vi "new_vi.vi"(6 "wait for reply (T)":bool=TRUE, 8 "error in":errorcluster) -> (0 "error out":errorcluster, 1 "timed out?":bool, 2 "result":string, 3 "vi_id":i32)   [LabVIEW 2025, in "Scripting Server.lvlib"]
doc: "Creates a new VI in the LabVIEW IDE. The VI Reference is stored and returned. This Reference can later be used to e.g. add modifications to the VI."
uses:
  Scripting Server.lvlib
  New VI Argument--cluster.ctl
  New VI (Reply Payload)--cluster.ctl
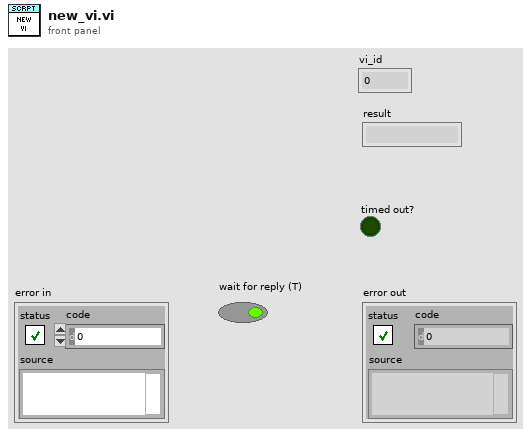
[diagram p1: front panel]
types:
  T1 = typedef "Scripting Server.lvlib/New VI Argument--cluster.ctl" = cluster{"Open Frontpanel":bool, "Wait Notifier":refnum<notifier>, "wait for reply":bool}
  T2 = typedef "Scripting Server.lvlib/Request Events--cluster.ctl" = cluster{"Stop Module":refnum<user-event>, "Show Panel":refnum<user-event>, "Hide Panel":refnum<user-event>, "Get Module Execution Status":refnum<user-event>, "Show Diagram":refnum<user-event>, "New VI":refnum<user-event>, "Add Object":refnum<user-event>, "Connect Objects":refnum<user-event>, "Get Object Terminals":refnum<user-event>, "get vi error list":refnum<user-event>, "Cleanup VI":refnum<user-event>, "create_control":refnum<user-event>, "Run VI":refnum<user-event>}
  T3 = typedef "Scripting Server.lvlib/New VI (Reply Payload)--cluster.ctl" = cluster{"VI Reference":i32, "Result":string, "error":errorcluster}
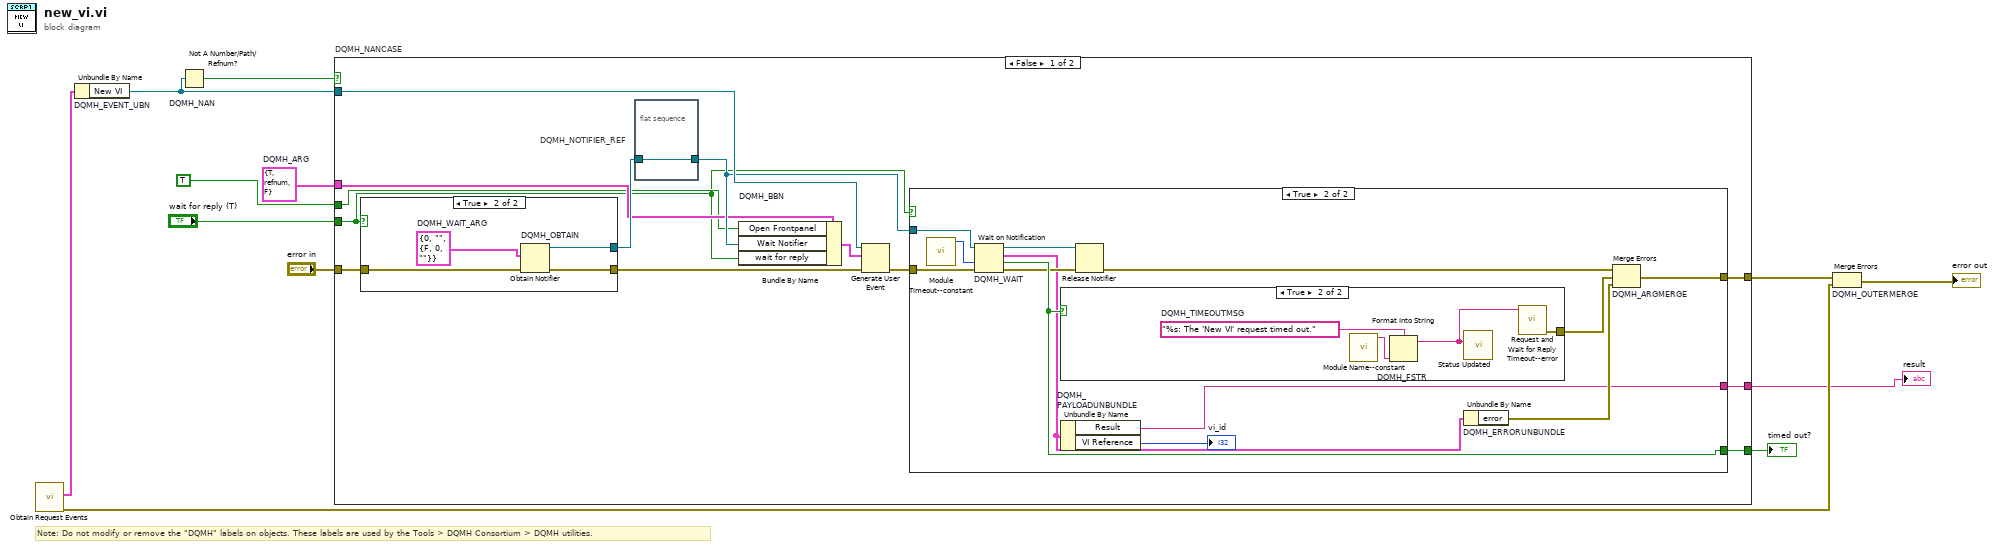
[diagram p0: block diagram]
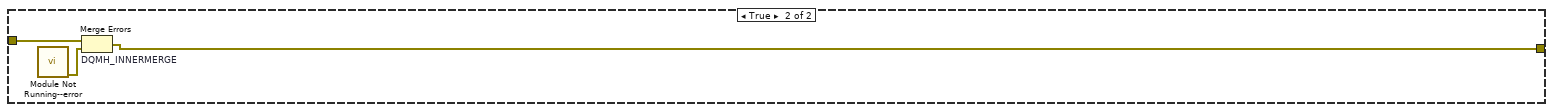
[diagram p5: hidden frame]
diagram:
  w6 = T1 {"Open Frontpanel"=TRUE, "Wait Notifier"=refnum, "wait for reply"=FALSE}  # DQMH_ARG
  # "Note: Do not modify or remove the \"DQMH\" labels on objects. These labels are used by the Tools > DQMH Consortium > DQMH utilities."
  n1 = call "Obtain Request Events.vi"() -> ("error out"=w3:errorcluster, "Scripting Server Request Events"=w2:T2)  [unwired: 10 in]
  n2 = Unbundle By Name "DQMH_EVENT_UBN"(w2) -> ("New VI"=w10:refnum<user-event>)
  n3 = Not A Number/Path/Refnum? "DQMH_NAN"(number/path/refnum=w10) -> (NaN/Path/Refnum?=w9:bool)
  n4 = case "DQMH_NANCASE" shown="False" w9 {
    tunnel: "error in" -> [w25 w52]
    tunnel: w10 -> [w23 _]
    tunnel: [w20 w51] -> w7
    tunnel: [w21 _] -> w8
    tunnel: w6 -> [w16 _]
    tunnel: TRUE ("open_frontpanel") -> [w15 _]
    tunnel: "wait for reply (T)" -> [w14 _]
    tunnel: [w13 _] -> w1
    frame False {
      n5 = case shown="True" w14 {
        tunnel: w25 -> [w45 w49]
        tunnel: [w45 w48] -> w22
        tunnel: [_ w46] -> w18
        frame False {
        }
        frame True {
          w47 = T3 {"VI Reference"=0, "Result"="", "error"={"status"=FALSE, "code"=0, "source"=""}}  # DQMH_WAIT_ARG
          n6 = Obtain Notifier "DQMH_OBTAIN"(notification data type=w47, error in (no error)=w49) -> (notifier out=w46:refnum<notifier>, error out=w48:errorcluster)  [unwired: 2 in, 1 out]
        }
      }
      n7 = flat-sequence "DQMH_NOTIFIER_REF" {
        tunnel: w18 -> [w26]
        tunnel: [w26] -> w17
        frame #0 {
        }
      }
      n8 = Bundle By Name "DQMH_BBN"(cluster=w16, "Open Frontpanel"=w15, "Wait Notifier"=w17, "wait for reply"=w14) -> (w19:T1)
      n9 = Generate User Event(user event=w23, event data cluster=w19, error in=w22) -> (error out=w24:errorcluster)  [unwired: 1 in, 1 out]
      n10 = case shown="True" w14 {
        tunnel: w24 -> [w27 w40]
        tunnel: w17 -> [_ w39]
        tunnel: [_ w37] -> w21
        tunnel: [w27 w36] -> w20
        tunnel: [_ w29] -> w13
        frame False {
        }
        frame True {
          n11 = call "Module Timeout--constant.vi"() -> ("Module Timeout"=w30:i32)  [unwired: 11 in]
          n12 = Wait on Notification "DQMH_WAIT"(notifier=w39, timeout in ms (-1)=w30, error in (no error)=w40) -> (notifier out=w38:refnum<notifier>, notification=w31:T3, timed out?=w37:bool, error out=w35:errorcluster)  [unwired: 1 in]
          n13 = case shown="True" w37 {
            tunnel: [_ w42] -> w32
            frame False {
            }
            frame True {
              w44 = "%s: The 'New VI' request timed out."  # DQMH_TIMEOUTMSG
              n14 = call "Module Name--constant.vi"() -> ("Module Name"=w41:string)  [unwired: 11 in]
              n15 = Format Into String "DQMH_FSTR"(format string=w44, w41) -> (resulting string=w43:string)  [unwired: 2 in, 1 out]
              n16 = call "Status Updated.vi"("Status"=w43) -> ()  [unwired: 10 in, 1 out]
              n17 = call "Request and Wait for Reply Timeout--error.vi"("Error Message"=w43) -> ("error out"=w42:errorcluster)  [unwired: 10 in]
            }
          }
          n18 = Unbundle By Name "DQMH_PAYLOADUNBUNDLE"(w31) -> ("Result"=w29:string, "VI Reference"=→"vi_id":i32)
          n19 = Release Notifier(notifier=w38, error in (no error)=w35) -> (error out=w34:errorcluster)  [unwired: 1 in, 2 out]
          n20 = Unbundle By Name "DQMH_ERRORUNBUNDLE"(w31) -> ("error"=w33:errorcluster)
          n21 = Merge Errors "DQMH_ARGMERGE"(w34, w32, w33) -> (w36:errorcluster)
        }
      }
    }
    frame True {
      n22 = call "Module Not Running--error.vi"() -> ("error out"=w50:errorcluster)  [unwired: 11 in]
      n23 = Merge Errors "DQMH_INNERMERGE"(w52, w50) -> (w51:errorcluster)
    }
  }
  "timed out?" <- w8
  "result" <- w1
  n24 = Merge Errors "DQMH_OUTERMERGE"(w7, w3) -> (→"error out":errorcluster)
